vi "usrp get time last pps.vi"(7 "frac_secs_out":dbl, 8 "error in (no error)":errorcluster, 9 "full_secs_out":i64, 10 "mboard":u64, 11 "h":u64) -> (0 "error out":errorcluster, 1 "full_secs_out out":i64, 3 "function return":u32(ring), 5 "frac_secs_out out":dbl)   [LabVIEW 2023, in "uhd.lvlib"]
doc: "UHD_API uhd_error uhd_usrp_get_time_last_pps(\n uhd_usrp_handle h, size_t mboard, int64_t* full_secs_out, double* frac_secs_out);"
uses:
  <userlib>/uhd/uhd.lvlib
  <userlib>/uhd/uhd.dll
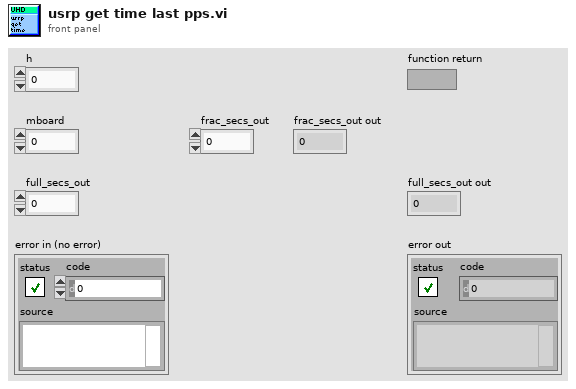
[diagram p1: front panel]
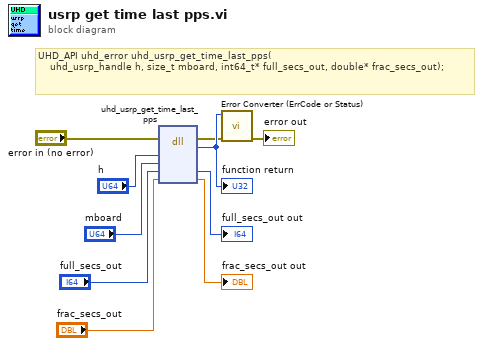
[diagram p0: block diagram]
diagram:
  # "UHD_API uhd_error uhd_usrp_get_time_last_pps(\n    uhd_usrp_handle h, size_t mboard, int64_t* full_secs_out, double* frac_secs_out);"
  n1 = dll-call lib="C:/Program Files/National Instruments/LabVIEW 2023/user.lib/uhd/uhd.*" fn="uhd_usrp_get_time_last_pps"(error in="error in (no error)", "h"="h", "mboard"="mboard", "full_secs_out"="full_secs_out", "frac_secs_out"="frac_secs_out") -> (error out=w2:errorcluster, w10:u32, "full_secs_out"=→"full_secs_out out":i64, "frac_secs_out"=→"frac_secs_out out":dbl)  [unwired: 4 in, 1 out]
  "function return" <- w10
  n2 = call <userlib>:"Error Converter (ErrCode or Status).vi"("error in (no error)"=w2, "error code"=w10) -> ("error out"=→"error out":errorcluster)  [unwired: 9 in]
